vi "BDR.vi"(0 "System no.":i32=1 min=1 step=1, 3 "Baudrate":dbl=57.6 format="%.4f", 4 "No. of digits":i16=1, 5 "error in":errorcluster) -> (19 "error out":errorcluster)   [LabVIEW 2026]
doc: "Set baud rate for RS-232 communication. Valid baud rates are 9.6, 19.2, 38.4, 57.6 and 115.2 (GCS 1.0) and 9600, 19200, 38400, 57600, 115200 (GCS 2.0). No. of digits is the number of digits after the decimal point in the baud rate specification that will be sent. VI waits 3 sec after sending BDR.\n\nE-755: No. of digits must be 0. Baudrate is given in baud. Baud rate changes with BDR.vi are done in RAM only. After the baud rate was changed with BDR.vi, Close connection if open.vi with Close Daisychain? = TRUE must be called and communications must be re-established with the new baud rate (see instruction in E-755 user manual). Incorrect entries may have unpredictable results and may not set an error status. Use WPA.vi to write the current baud rate setting to non-volatile memory where it becomes the power-on default. Check RAM setting with BDR?.vi before running WPA.vi. \n\nE-816: No. of digits must be 1. Baudrate is given in kbaud. Baudrate changes must be written to non-volatile memory with WPA.vi and do not take effect before the next power on or RST. Incorrect entries (such as 56) have unpredictable results and may not set an error status. Check RAM setting with BDR?.vi after setting the baudrate before running WPA.vi. This command cannot be issued to a slave E-816."
panel:
  # "Set baudrate for RS-232 communication. Valid baudrates\nare 9.6, 19.2, 38.4, 57.6 and 115.2 (GCS 1.0) and 9600, 19200, 38400, 57600, 115200 (GCS 2.0). VI waits 3 sec after sending BDR."
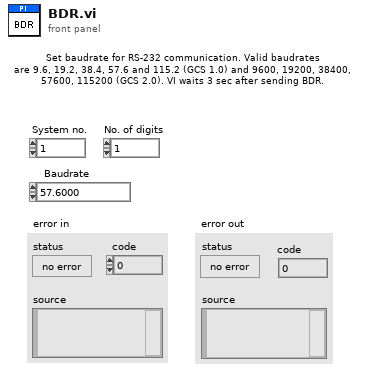
[diagram p1: front panel]
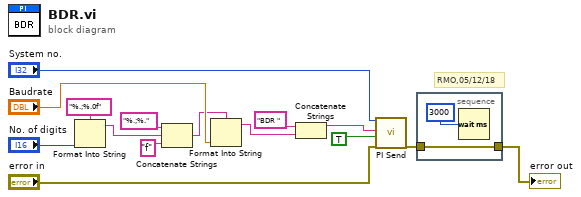
[diagram p0: block diagram]
diagram:
  # "RMO,05/12/18"
  n1 = Format Into String(format string="%.;%.0f" ("Format String"), "No. of digits") -> (resulting string=w4:string)  [unwired: 2 in, 1 out]
  n2 = Concatenate Strings("%.;%." ("Format String"), w4, "f" ("Format String")) -> (w2:string)
  n3 = Format Into String(format string=w2, "Baudrate") -> (resulting string=w9:string)  [unwired: 2 in, 1 out]
  n4 = Concatenate Strings("BDR ", w9) -> (w11:string)
  n5 = call "PI Send.vi"("System no."="System no.", "String to send"=w11, "Attach termination char.?"=TRUE ("Attach Linefeed?"), "error in"="error in") -> ("error out"=w8:errorcluster)  [unwired: 2 in, 13 out]
  n6 = stacked-sequence {
    tunnel: w8 -> [w16]
    tunnel: [w16] -> w1
    frame #0 {
      n7 = Wait (ms)(milliseconds to wait=u32 3000 ("millisecond timer value")) -> ()  [unwired: 1 out]
    }
  }
  "error out" <- w1
